vi "test-TimeInterpDouble-Test2.vi"() -> (3 "All tests passed":bool)   [LabVIEW 2019]
uses:
  <vilib>/Rock Robotics/WPI/ThirdParty/JAS_Junk/TrajLib/TimeInterpDouble_CleanUp.vi
  <vilib>/gmath/interp.llb/Search Ordered Table.vi
  <vilib>/Rock Robotics/WPI/ThirdParty/JAS_Junk/TrajLib/Trajectory_Library.lvlib
panel:
  out "Add Error":bool
  out "Error 1":bool
  out "Error 2":bool
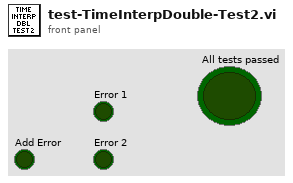
[diagram p1: front panel]
types:
  T1 = typedef "Trajectory_Library.lvlib/TIME_INTERPOLATABLE_DOUBLE.ctl" = cluster{"TimeStamps":dbl[], "DoubleValue":dbl[], "Min_TimeStamp":dbl, "Max_TimeStamp":dbl, "ItemCount":i32, "MaxBufferTime":dbl}
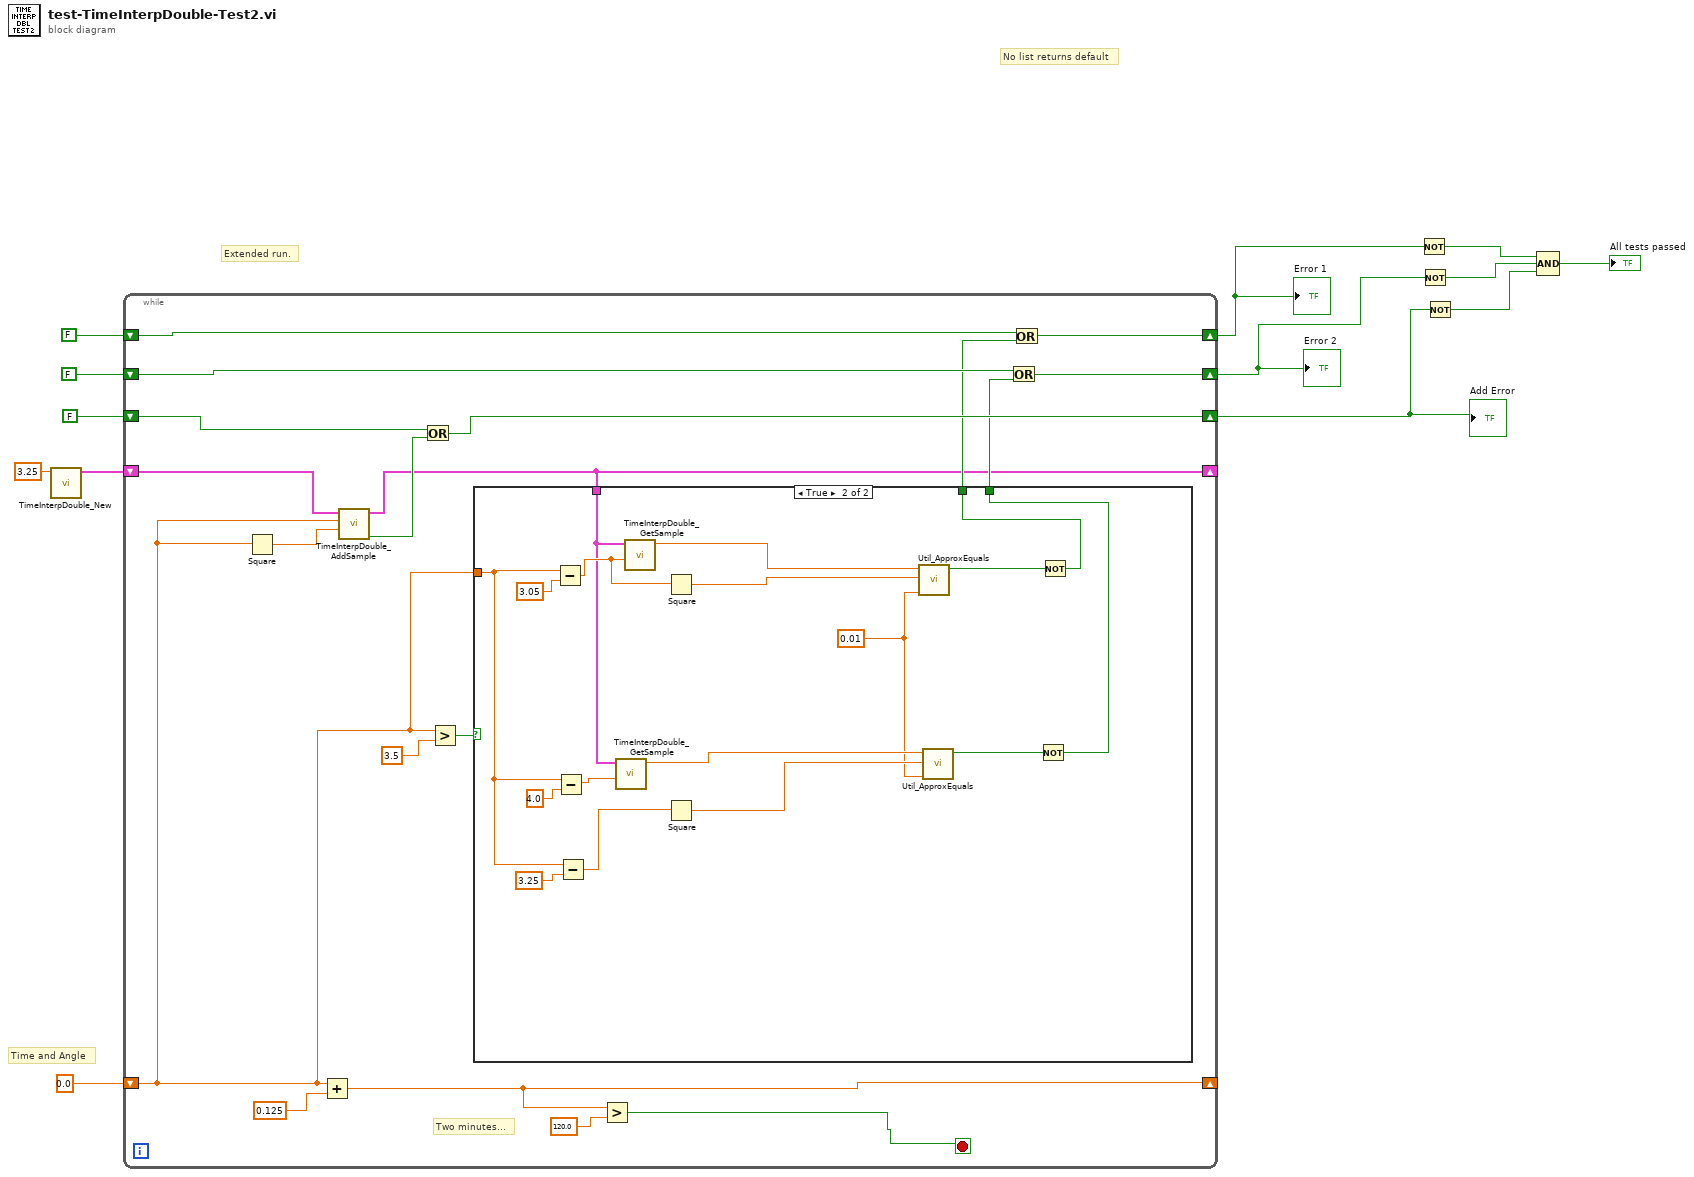
[diagram p0: block diagram]
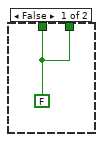
[diagram p2: hidden frame]
diagram:
  # "Extended run."
  # "Time and Angle"
  # "No list returns default"
  n1 = call <vilib>:"TimeInterpDouble_New.vi"("MaxTime"=3.25) -> ("TimeInterpDouble"=w11:T1)  [unwired: 10 in]
  n2 = while {
    shift-right: [w29] -> _
    shift-left: 0.0 -> [w16]
    shift-right: [w14] -> _
    shift-left: w11 -> [w15]
    shift-right: [w22] -> w7
    shift-left: FALSE -> [w27]
    shift-right: [w23] -> w5
    shift-left: FALSE -> [w20]
    shift-right: [w24] -> w6
    shift-left: FALSE -> [w21]
    stop <- w32 stop-if-true
    # "Two minutes..."
    n3 = Square(x=w16) -> (x^2=w17:dbl)
    n4 = Add(x=w16, y=0.125) -> (x+y=w29:dbl)
    n5 = call <vilib>:"TimeInterpDouble_AddSample.vi"("Value"=w17, "TimeStamp"=w16, "in TimeInterpDouble"=w15) -> ("Error"=w28:bool, "out TimeInterpDouble"=w14:T1)  [unwired: 7 in]
    n6 = Or(x=w27, y=w28) -> (x .or. y?=w22:bool)
    n7 = Greater?(x=w16, y=3.5) -> (0:w26:bool)
    n8 = case shown="True" w26 {
      tunnel: w16 -> [_ w47]
      tunnel: [w33 w45] -> w19
      tunnel: [w33 w44] -> w18
      tunnel: w14 -> [_ w41]
      frame False {
        w33 = FALSE
      }
      frame True {
        w35 = 0.01 ("Tolerance")
        n9 = Subtract(x=w47, y=3.05) -> (x-y=w42:dbl)
        n10 = Subtract(x=w47, y=4.0) -> (x-y=w49:dbl)
        n11 = Subtract(x=w47, y=3.25) -> (x-y=w37:dbl)
        n12 = call <vilib>:"TimeInterpDouble_GetSample.vi"("TimeStamp"=w49, "TimeInterpDouble"=w41) -> ("OutputDouble"=w38:dbl)  [unwired: 9 in]
        n13 = call <vilib>:"TimeInterpDouble_GetSample.vi"("TimeStamp"=w42, "TimeInterpDouble"=w41) -> ("OutputDouble"=w34:dbl)  [unwired: 9 in]
        n14 = Square(x=w42) -> (x^2=w40:dbl)
        n15 = Square(x=w37) -> (x^2=w36:dbl)
        n16 = call <vilib>:"Util_ApproxEquals.vi"("Tolerance"=w35, "Value 2"=w40, "Value 1"=w34) -> ("ApproxEquals"=w43:bool)  [unwired: 8 in]
        n17 = call <vilib>:"Util_ApproxEquals.vi"("Tolerance"=w35, "Value 2"=w36, "Value 1"=w38) -> ("ApproxEquals"=w39:bool)  [unwired: 8 in]
        n18 = Not(x=w39) -> (.not. x?=w44:bool)
        n19 = Not(x=w43) -> (.not. x?=w45:bool)
      }
    }
    n20 = Greater?(x=w29, y=120.0) -> (0:w32:bool)
    n21 = Or(x=w20, y=w18) -> (x .or. y?=w23:bool)
    n22 = Or(x=w21, y=w19) -> (x .or. y?=w24:bool)
  }
  "Add Error" <- w7
  "Error 1" <- w6
  "Error 2" <- w5
  n23 = Not(x=w6) -> (.not. x?=w4:bool)
  n24 = Not(x=w5) -> (.not. x?=w3:bool)
  n25 = Not(x=w7) -> (.not. x?=w2:bool)
  n26 = Compound Arithmetic op=AND(w4, w3, w2) -> (→"All tests passed":bool)
